vi "GetDVRref.vi"(8 "error in (no error)":errorcluster, 10 "data value reference":refnum<data-value>, 11 "Add in":refnum<class "Add.lvclass">) -> (0 "error out":errorcluster, 1 "Arithmetic out":refnum<class "Arithmetic.lvclass">, 2 "data value reference":refnum<data-value>, 3 "Add out":refnum<class "Add.lvclass">)   [LabVIEW 2023, in "Add.lvclass"]
uses:
  Add.lvclass
  Arithmetic/Arithmetic.lvclass
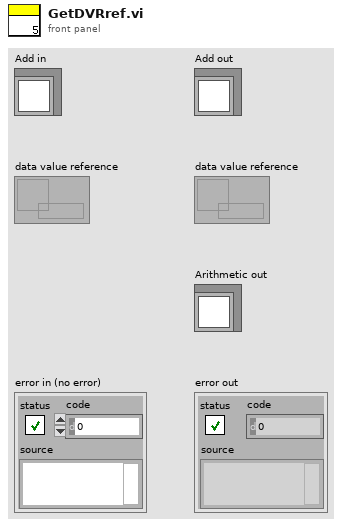
[diagram p1: front panel]
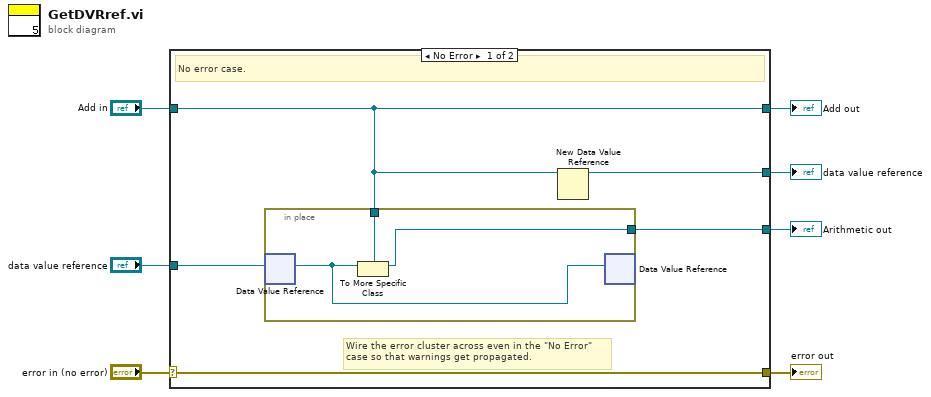
[diagram p0: block diagram]
diagram:
  n1 = case shown="No Error" "error in (no error)" {
    selector: "error in (no error)" -> [w12 w17]
    tunnel: [w12 w17] -> w6
    tunnel: [w9 w16] -> w4
    tunnel: "Add in" -> [w9 w16]
    tunnel: [w11 _] -> w3
    tunnel: "data value reference" -> [w10 _]
    tunnel: [w8 _] -> w1
    frame No Error {
      # "Wire the error cluster across even in the \"No Error\"\ncase so that warnings get propagated."
      # "No error case."
      n2 = in-place {
        in-place-border: w9 -> [w15]
        in-place-border: [w14] -> w8
        n3 = in-place-dvr #1(w10) -> (w13:refnum<class "Arithmetic.lvclass">)  [unwired: 1 out]
        n4 = To More Specific Class(target class=w15, reference=w13) -> (specific class reference=w14:refnum<class "Add.lvclass">)  [unwired: 1 in, 1 out]
        n5 = in-place-dvr #1(w13) -> ()  [unwired: 2 out]
      }
      n6 = New Data Value Reference(data value=w9) -> (data value reference=w11:refnum<data-value>)  [unwired: 1 in, 1 out]
    }
    frame Error {
      # "No error case."
    }
  }
  "error out" <- w6
  "Add out" <- w4
  "data value reference" <- w3
  "Arithmetic out" <- w1
